vi "[FJC] Calculate Contour Length.vi"(1 "Temperature (K)":dbl=298.0, 2 "Force (pN)":dbl, 3 "Segment Length (nm)":dbl, 4 "Segment Elasticity (pN/nm)":dbl, 5 "Persistence Length (nm)":dbl, 6 "Extension (nm)":dbl) -> (0 "Contour Length (nm)":dbl)   [LabVIEW 2013]
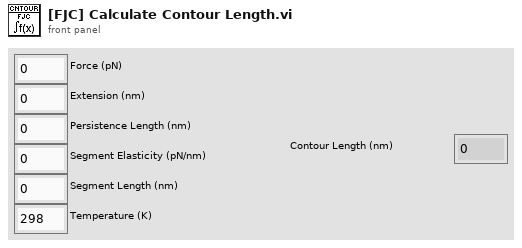
[diagram p1: front panel]
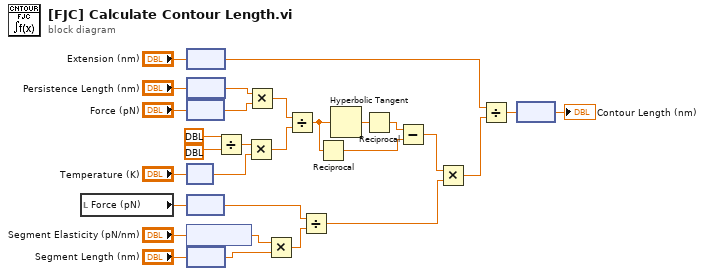
[diagram p0: block diagram]
diagram:
  n1 = local read "Force (pN)"() -> (w13:dbl)
  n2 = node("Extension (nm)") -> (w6:dbl[unit])
  n3 = node("Persistence Length (nm)") -> (w26:dbl[unit])
  n4 = node("Force (pN)") -> (w25:dbl[unit])
  n5 = node("Temperature (K)") -> (w21:dbl[unit])
  n6 = node(w13) -> (w11:dbl[unit])
  n7 = node("Segment Elasticity (pN/nm)") -> (w15:dbl[unit])
  n8 = node("Segment Length (nm)") -> (w14:dbl[unit])
  n9 = Divide(x=ext[unit] 8.314472, y=ext[unit] 6.0221415e+23) -> (x/y=w23:ext[unit])
  n10 = Multiply(x=w23, y=w21) -> (x*y=w18:ext[unit])
  n11 = Multiply(x=w26, y=w25) -> (x*y=w19:dbl[unit])
  n12 = Multiply(x=w15, y=w14) -> (x*y=w12:dbl[unit])
  n13 = Divide(x=w19, y=w18) -> (x/y=w2:ext)
  n14 = Divide(x=w11, y=w12) -> (x/y=w7:dbl)
  n15 = Reciprocal(x=w2) -> (1/x=w9:ext)
  n16 = Hyperbolic Tangent(1:w2) -> (0:w1:ext)
  n17 = Reciprocal(x=w1) -> (1/x=w10:ext)
  n18 = Subtract(x=w10, y=w9) -> (x-y=w8:ext)
  n19 = Multiply(x=w8, y=w7) -> (x*y=w5:ext)
  n20 = Divide(x=w6, y=w5) -> (x/y=w4:ext[unit])
  n21 = node(w4) -> (→"Contour Length (nm)":ext)
